vi "GetText.vi"(8 "error in":errorcluster, 11 "Temperature Chamber Model editor node in":refnum<class "Temperature Chamber Model editor node.lvclass">) -> (0 "error out":errorcluster, 1 "additional text":string, 2 "text":string, 3 "Temperature Chamber Model editor node out":refnum<class "Temperature Chamber Model editor node.lvclass">, 4 "glyph":string)   [LabVIEW 2013, in "Temperature Chamber Model editor node.lvclass"]
uses:
  Temperature Chamber Model editor node.lvclass
  <vilib>/NI/Tag Bus Data Framework/Configuration Editor/subVIs/Glyphs Status.ctl
  <vilib>/NI/Tag Bus Data Framework/fixed module parent/editor node/fixed channel editor.lvclass
  <vilib>/NI/Tag Bus Data Framework/Configuration Editor/PL Framework Configuration Tool.lvlib
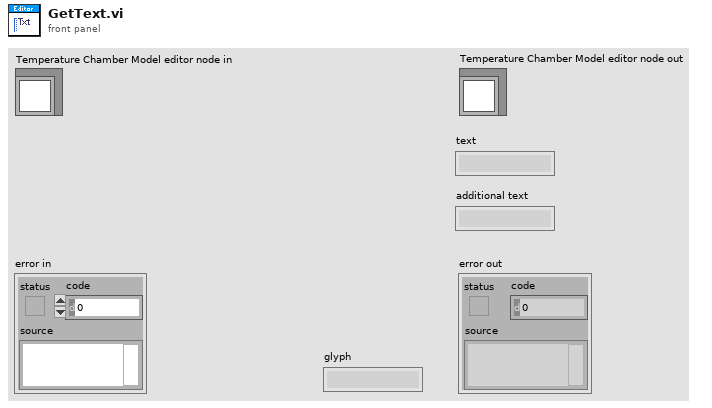
[diagram p1: front panel]
types:
  T1 = typedef "PL Framework Configuration Tool.lvlib/Glyphs Status.ctl" = enum16{"Normal", "Error"}
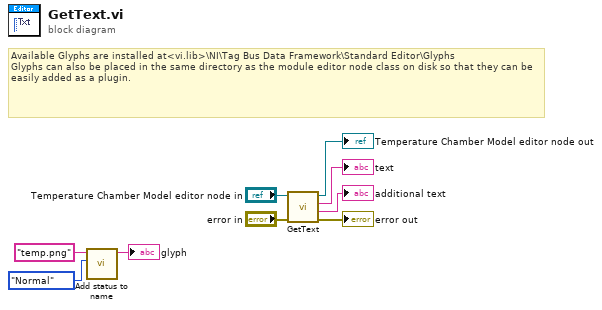
[diagram p0: block diagram]
diagram:
  # "Available Glyphs are installed at<vi.lib>\\NI\\Tag Bus Data Framework\\Standard Editor\\Glyphs\nGlyphs can also be placed in the same directory as the module editor node class on disk so that they can be easily added as a plugin."
  n1 = call <vilib>:"Add status to name.vi"("Status"=Glyphs_Status."Normal", "Name"="temp.png" ("glyph")) -> ("Name with status"=→"glyph":string)  [unwired: 9 in]
  n2 = call-parent "GetText.vi"("error in"="error in", "Module Editor Node in"="Temperature Chamber Model editor node in") -> ("error out"=→"error out":errorcluster, "additional text"=→"additional text":string, "text"=→"text":string, "Module Editor Node out"=→"Temperature Chamber Model editor node out":refnum<class "Temperature Chamber Model editor node.lvclass">)  [unwired: 5 in, 1 out]
